vi "Cell Photo.vi"(10 "Serial Number":string="1234", 11 "Part Number":string="B0CG1KL3RC") -> (0 "error out":errorcluster, 2 "File ID":string, 3 "Image Path":string)   [LabVIEW 2024]
uses:
  <vilib>/Skyline/File/HTTP/Send File HTTP.vi
  <vilib>/Skyline/File/HTTP/NI Skyline File HTTP.lvclass
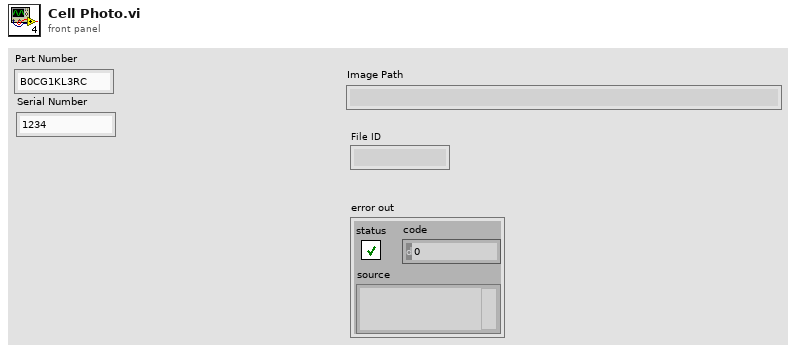
[diagram p1: front panel]
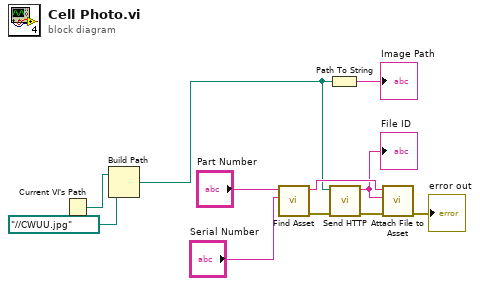
[diagram p0: block diagram]
diagram:
  n1 = Current VI's Path() -> (path=w3:path)
  n2 = Build Path(base path=w3, name or relative path=path "../../CWUU.jpg") -> (appended path=w1:path)
  n3 = call "Find Asset.vi"("Serial Number"="Serial Number", "Part Number"="Part Number") -> ("error out"=w7:errorcluster, "Asset ID"=w8:string)  [unwired: 7 in, 1 out]
  n4 = Path To String(path=w1) -> (string=→"Image Path":string)
  n5 = call-poly <vilib>:"Send HTTP.vi"("error in (no error)"=w7, "path"=w1) -> ("error out"=w6:errorcluster, "id"=w5:string)  [unwired: 7 in]
  "File ID" <- w5
  n6 = call "Attach File to Asset.vi"("error in (no error)"=w6, "File ID"=w5, "Asset ID"=w8) -> ("error out"=→"error out":errorcluster)  [unwired: 8 in]
